vi "GetBarcode 2DResultNames.vi"(7 "ProjectName":string="Prj", 10 "data IN":T1={"ROI"={"Global Rectangle"=[], "Contours"=[]}, "Barcode Type"=enum."PDF417", "Data Matrix Parameter"={"Data Matrix Description Options"={"Aspect Ratio"=0.0, "Rows"=0, "Columns"=0, "Rectangle"=FALSE, "ECC"=-2, "Barcode Polarity"=0, "Cell Fill Percentage"=-2, "Minimum Border Integrity %"=80.0, "Mirror Mode"=-2}, "Data Matrix Search Options"={"Rotation Mode"=enum."Unlimited", "Skip Location?"=FALSE, "Edge Threshold"=30, "Demodulation Mode"=-2, "Cell Sample Size"=-2, "Cell Filter Mode"=-2, "Skew Degrees Allowed"=5, "Maximum Iterations"=500, "Initial Search Vector Width"=5}, "Data Matrix Size Options"={"Data Matrix Size"={"Minimum Size"=0, "Maximum Size"=0}, "Quiet Zone Width"=10}, "Advanced Options"=[]}, "PDF147 Search Mode"=enum."Multiple Barcodes", "QR Code Parameter"={"QR Search Options"={"Rotation Mode"=enum."Unlimited", "Skip Location?"=FALSE, "Edge Threshold"=30, "Demodulation Mode"=-2, "Cell Sample Size"=-2, "Cell Filter Mode"=-2, "Skew Degrees Allowed"=5}, "QR Description Options"={"Matrix Size (cells)"=0, "Barcode Polarity"=-2, "Mirror Mode"=-2, "QR Model"=0}, "QR Code Cell Size (pixels)"={"Minimum Size"=3, "Maximum Size"=7}}} {"QR Code Parameter"."QR Description Options"."Mirror Mode" items=["Auto-detect"=-2, "Normal"=0, "Mirrored"=1]; "QR Code Parameter"."QR Description Options"."Matrix Size (cells)" items=["Auto-detect"=0, "11x11 - Version 1 (Micro QR Only)"=11, "13x13 - Version 2 (Micro QR Only)"=13, "15x15 - Version 3 (Micro QR Only)"=15, "17x17 - Version 4 (Micro QR Only)"=17, "21x21 - Version 1"=21, "25x25 - Version 2"=25, "29x29 - Version 3"=29, "33x33 - Version 4"=33, "37x37 - Version 5"=37, "41x41 - Version 6"=41, "45x45 - Version 7"=45, "49x49 - Version 8"=49, "53x53 - Version 9"=53, "57x57 - Version 10"=57, "61x61 - Version 11"=61, "65x65 - Version 12"=65, "69x69 - Version 13"=69, "73x73 - Version 14"=73, "77x77 - Version 15"=77, "81x81 - Version 16"=81, "85x85 - Version 17"=85, "89x89 - Version 18"=89, "93x93 - Version 19"=93, "97x97 - Version 20"=97, "101x101 - Version 21"=101, "105x105 - Version 22"=105, "109x109 - Version 23"=109, "113x113 - Version 24"=113, "117x117 - Version 25"=117, "121x121 - Version 26"=121, "125x125 - Version 27"=125, "129x129 - Version 28"=129, "133x133 - Version 29"=133, "137x137 - Version 30"=137, "141x141 - Version 31"=141, "145x145 - Version 32"=145, "149x149 - Version 33"=149, "153x153 - Version 34"=153, "157x157 - Version 35"=157, "161x161 - Version 36"=161, "165x165 - Version 37"=165, "169x169 -  Version 38"=169, "173x173 - Version 39"=173, "177x177 - Version 40"=177]; "QR Code Parameter"."QR Description Options"."QR Model" items=["Auto-detect", "Micro", "Model 1", "Model 2"]; "QR Code Parameter"."QR Description Options"."Barcode Polarity" items=["Auto-detect"=-2, "Black on White"=0, "White on Black"=1]; "QR Code Parameter"."QR Search Options"."Cell Filter Mode" items=["Auto-detect"=-2, "Average"=0, "Median"=1, "Central Average"=2, "High Average"=3, "Low Average"=4, "Very High Average"=5, "Very Low Average"=6, "All Filters"=8]; "QR Code Parameter"."QR Search Options"."Cell Sample Size" items=["Auto-detect"=-2, "1x1"=1, "2x2"=2, "3x3"=3, "4x4"=4, "5x5"=5, "6x6"=6, "7x7"=7]; "QR Code Parameter"."QR Search Options"."Demodulation Mode" items=["Auto-detect"=-2, "Histogram"=0, "Local Contrast"=1, "Combination"=2, "All"=3]; "Data Matrix Parameter"."Advanced Options"."Value" format="%.2f"; "Data Matrix Parameter"."Data Matrix Search Options"."Cell Filter Mode" items=["Auto-detect"=-2, "Average"=0, "Median"=1, "Central Average"=2, "High Average"=3, "Low Average"=4, "Very High Average"=5, "Very Low Average"=6, "All Filters"=8]; "Data Matrix Parameter"."Data Matrix Search Options"."Cell Sample Size" items=["Auto-detect"=-2, "1x1"=1, "2x2"=2, "3x3"=3, "4x4"=4, "5x5"=5, "6x6"=6, "7x7"=7]; "Data Matrix Parameter"."Data Matrix Search Options"."Demodulation Mode" items=["Auto-detect"=-2, "Histogram"=0, "Local Contrast"=1, "Combination"=2, "All"=3]; "Data Matrix Parameter"."Data Matrix Description Options"."Mirror Mode" items=["Auto-detect"=-2, "Normal"=0, "Mirrored"=1]; "Data Matrix Parameter"."Data Matrix Description Options"."ECC" items=["Auto-detect"=-2, "ECC 000"=0, "ECC 050"=50, "ECC 080"=80, "ECC 100"=100, "ECC 140"=140, "ECC 000-140"=190, "ECC 200"=200]; "Data Matrix Parameter"."Data Matrix Description Options"."Minimum Border Integrity %" format="%.2f"; "Data Matrix Parameter"."Data Matrix Description Options"."Aspect Ratio" format="%.2f"; "Data Matrix Parameter"."Data Matrix Description Options"."Cell Fill Percentage" items=["Auto-detect"=-2, "< 30%"=0, ">= 30%"=1]; "Data Matrix Parameter"."Data Matrix Description Options"."Barcode Polarity" items=["Auto-detect"=-2, "Black on White"=0, "White on Black"=1]}, 11 "ROI_Name":string="ROI1") -> (3 "ResultNames":string[](array[string]))   [LabVIEW 2019]
uses:
  Controls/Barcode 2D/Analysis_Barcode 2D_Result.ctl
  <vilib>/vision/Instrument.llb/QR Code Report.ctl
  <vilib>/vision/Instrument.llb/QR Code Model Type.ctl
  <vilib>/vision/Instrument.llb/QR Code Stream Mode Type.ctl
  <vilib>/vision/Instrument.llb/Data Matrix Polarity.ctl
  <vilib>/vision/Instrument.llb/Demodulation Mode.ctl
  <vilib>/vision/Instrument.llb/Cell Sample Size.ctl
  <vilib>/vision/Instrument.llb/Cell Filter Mode.ctl
  Controls/Barcode 2D/Analysis_Barcode 2D_Parameter.ctl
  <vilib>/vision/Instrument.llb/Data Matrix Description Options.ctl
  <vilib>/vision/Instrument.llb/ECC Type.ctl
  <vilib>/vision/Instrument.llb/Cell Fill Percentage.ctl
  <vilib>/vision/Instrument.llb/Data Matrix Mirror.ctl
  <vilib>/vision/Instrument.llb/Data Matrix Search Options.ctl
  <vilib>/vision/Instrument.llb/Data Matrix Size Options.ctl
  <vilib>/vision/Instrument.llb/Data Matrix Advanced Options.ctl
  <vilib>/vision/Instrument.llb/QR Code Search Options.ctl
  <vilib>/vision/Instrument.llb/QR Code Description Options.ctl
panel:
  out "Analysis_Barcode 2D_Result":T17={"QR Code Report"={"Found?"=FALSE, "Data"="", "Bounding Box"=[], "Errors Corrected"=0, "Dimensions (Rows/Cols)"=0, "Version"=0, "QR Model"=0, "Stream Mode"=0, "Barcode Polarity"=-2, "Mirrored?"=FALSE, "Append Stream Position"=0, "Size of Append Stream"=0, "First EAN-128 ID"=0, "First Alternate Language ID"=0, "Append Stream ID"=0, "Minimum Edge Strength"=30, "Demodulation Mode"=-2, "Cell Sample Size"=-2, "Cell Filter Mode"=-2}} {"QR Code Report"."Append Stream ID" format="%x"; "QR Code Report"."Cell Filter Mode" items=["Auto-detect"=-2, "Average"=0, "Median"=1, "Central Average"=2, "High Average"=3, "Low Average"=4, "Very High Average"=5, "Very Low Average"=6, "All Filters"=8]; "QR Code Report"."Cell Sample Size" items=["Auto-detect"=-2, "1x1"=1, "2x2"=2, "3x3"=3, "4x4"=4, "5x5"=5, "6x6"=6, "7x7"=7]; "QR Code Report"."Demodulation Mode" items=["Auto-detect"=-2, "Histogram"=0, "Local Contrast"=1, "Combination"=2, "All"=3]; "QR Code Report"."Barcode Polarity" items=["Auto-detect"=-2, "Black on White"=0, "White on Black"=1]; "QR Code Report"."Stream Mode" items=["Numeric", "AlphaNumeric", "Raw Bytes", "UCC/EAN-128 - In Tokens", "UCC/EAN-128 - In Data", "Extended Character Interpretation", "Kanji"]; "QR Code Report"."QR Model" items=["Auto-detect", "Micro", "Model 1", "Model 2"]; "QR Code Report"."Version" max=40 step=1}
  out "error out":errorcluster
  in  "error in (no error)":errorcluster
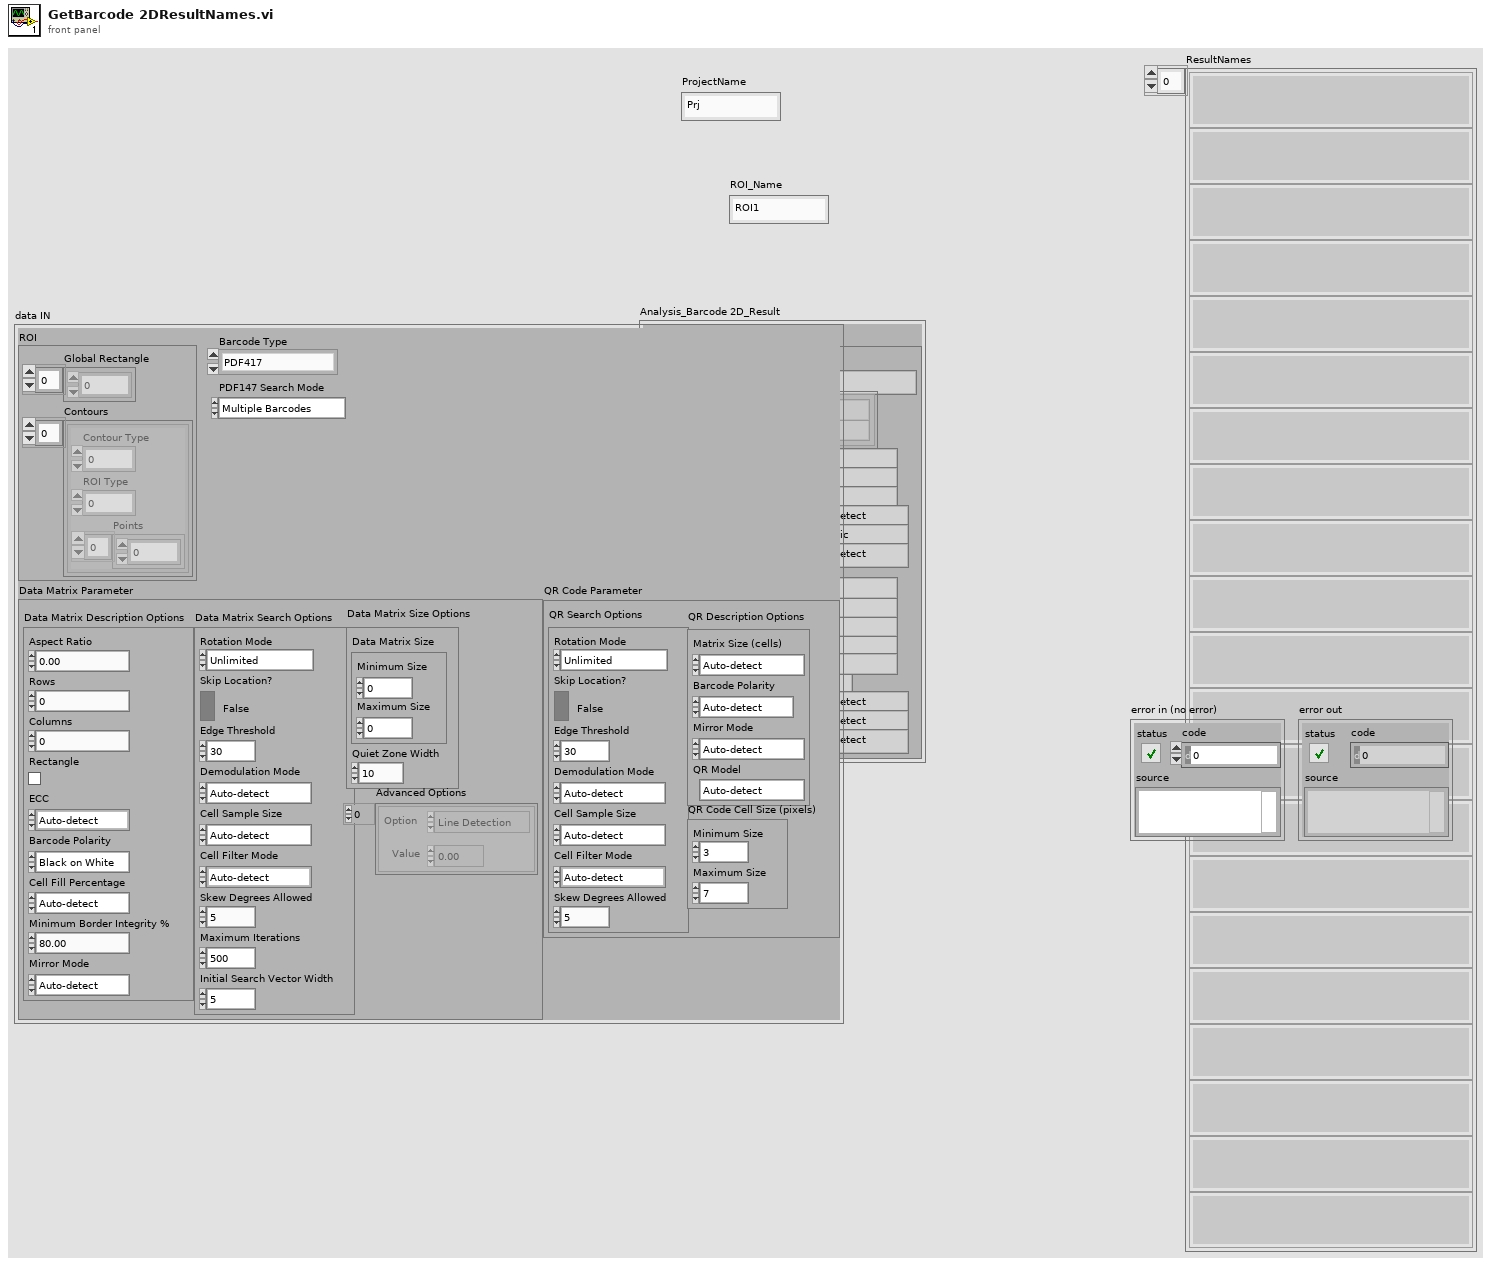
[diagram p1: front panel]
types:
  T1 = typedef "Analysis_Barcode 2D_Parameter.ctl" = cluster{"ROI":cluster{"Global Rectangle":i32[], "Contours":cluster{"Contour Type":u32, "ROI Type":u32, "Points":i32[]}[]}, "Barcode Type":enum16{"Data Matrix", "PDF417", "QR Code"}, "Data Matrix Parameter":cluster{"Data Matrix Description Options":T2, "Data Matrix Search Options":T7, "Data Matrix Size Options":T11, "Advanced Options":T12[]}, "PDF147 Search Mode":T13, "QR Code Parameter":cluster{"QR Search Options":T14, "QR Description Options":T15, "QR Code Cell Size (pixels)":cluster{"Minimum Size":u32, "Maximum Size":u32}}}
  T2 = typedef "Data Matrix Description Options.ctl" = cluster{"Aspect Ratio":sgl, "Rows":u32, "Columns":u32, "Rectangle":bool, "ECC":T3, "Barcode Polarity":T4, "Cell Fill Percentage":T5, "Minimum Border Integrity %":sgl, "Mirror Mode":T6}
  T3 = typedef "ECC Type.ctl" = i32
  T4 = typedef "Data Matrix Polarity.ctl" = i32
  T5 = typedef "Cell Fill Percentage.ctl" = i32
  T6 = typedef "Data Matrix Mirror.ctl" = i32
  T7 = typedef "Data Matrix Search Options.ctl" = cluster{"Rotation Mode":enum32{"Unlimited", "0 Degrees", "90 Degrees", "180 Degrees", "270 Degrees"}, "Skip Location?":bool, "Edge Threshold":u32, "Demodulation Mode":T8, "Cell Sample Size":T9, "Cell Filter Mode":T10, "Skew Degrees Allowed":u32, "Maximum Iterations":u32, "Initial Search Vector Width":u32}
  T8 = typedef "Demodulation Mode.ctl" = i32
  T9 = typedef "Cell Sample Size.ctl" = i32
  T10 = typedef "Cell Filter Mode.ctl" = i32
  T11 = typedef "Data Matrix Size Options.ctl" = cluster{"Data Matrix Size":cluster{"Minimum Size":u32, "Maximum Size":u32}, "Quiet Zone Width":u32}
  T12 = typedef "Data Matrix Advanced Options.ctl" = cluster{"Option":enum32{"Line Detection", "HighLight Filter", "Aggressive", "FNC1", "Refine Bounding Box"}, " Value":dbl}
  T13 = typedef "PDF417 Search Mode" = enum32{"Multiple Barcodes", "Single Barcode, Conservative"}
  T14 = typedef "QR Code Search Options.ctl" = cluster{"Rotation Mode":enum32{"Unlimited", "0 Degrees", "90 Degrees", "180 Degrees", "270 Degrees"}, "Skip Location?":bool, "Edge Threshold":u32, "Demodulation Mode":T8, "Cell Sample Size":T9, "Cell Filter Mode":T10, "Skew Degrees Allowed":u32}
  T15 = typedef "QR Code Description Options.ctl" = cluster{"Matrix Size (cells)":i32, "Barcode Polarity":T4, "Mirror Mode":i32, "QR Model":T16}
  T16 = typedef "QR Code Model Type.ctl" = i32
  T17 = typedef "Analysis_Barcode 2D_Result.ctl" = cluster{"QR Code Report":T18}
  T18 = typedef "QR Code Report.ctl" = cluster{"Found?":bool, "Data":string, "Bounding Box":cluster{"x":sgl, "y":sgl}[], "Errors Corrected":u32, "Dimensions (Rows/Cols)":u32, "Version":u32, "QR Model":T16, "Stream Mode":T19, "Barcode Polarity":T4, "Mirrored?":bool, "Append Stream Position":u32, "Size of Append Stream":u32, "First EAN-128 ID":i32, "First Alternate Language ID":i32, "Append Stream ID":u32, "Minimum Edge Strength":u32, "Demodulation Mode":T8, "Cell Sample Size":T9, "Cell Filter Mode":T10}
  T19 = typedef "QR Code Stream Mode Type.ctl" = i32
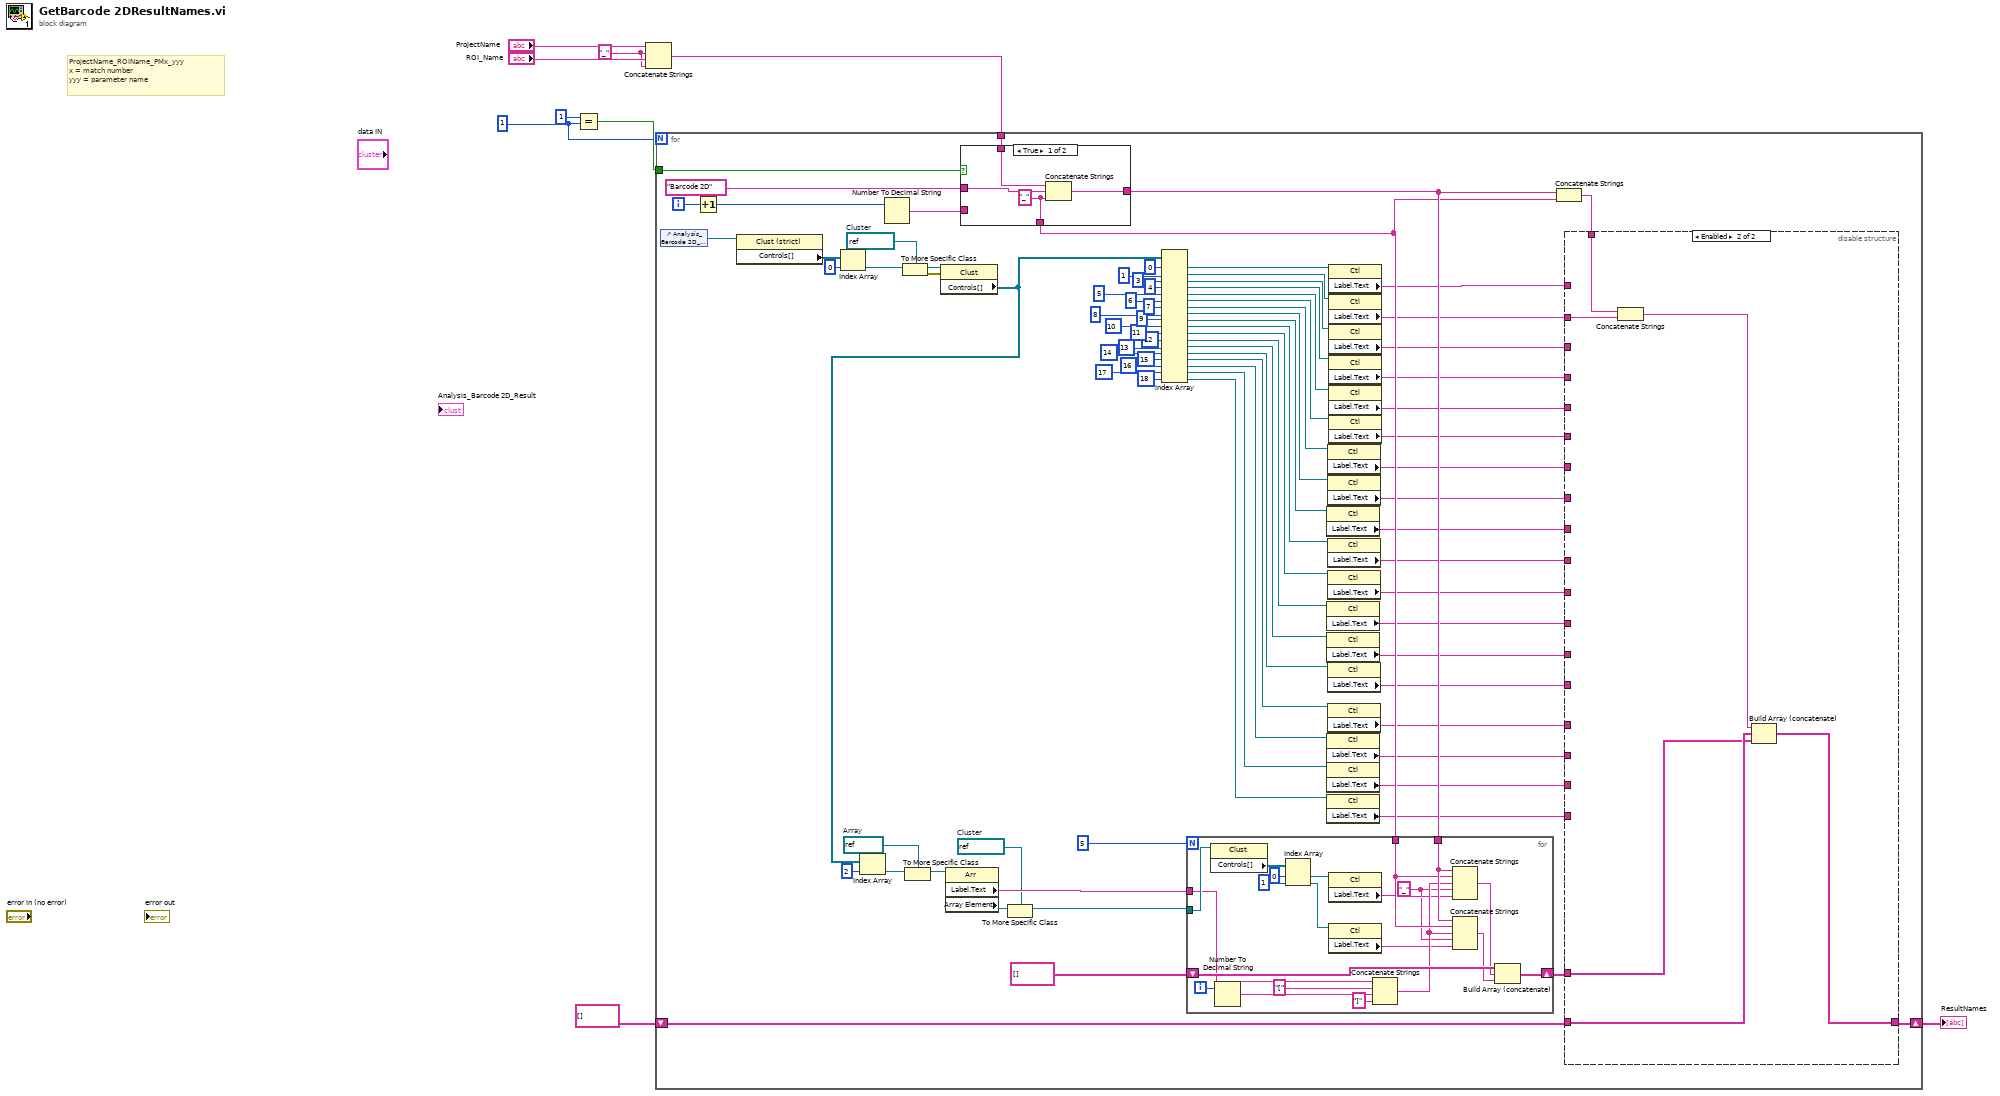
[diagram p0: block diagram]
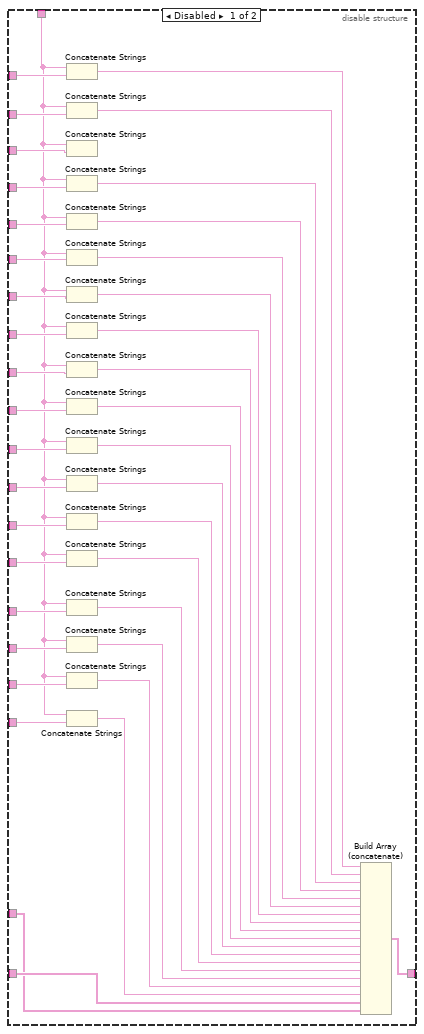
[diagram p2: hidden frame]
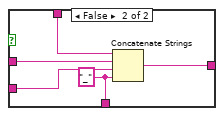
[diagram p3: hidden frame]
diagram:
  w1 = 1
  w6 = "_" ("string")
  # "ProjectName_ROIName_PMx_yyy\nx = match number\nyyy = parameter name"
  n1 = Equal?(x=1, y=w1) -> (x = y?=w2:bool)
  n2 = Concatenate Strings("ProjectName", w6, "ROI_Name", w6) -> (w5:string)
  n3 = for {
    N: w1 -> [_]
    tunnel: w5 -> [w91]
    shift-right: [w64] -> w3
    shift-left: string[] [] -> [w87]
    tunnel: w2 -> [w92]
    i -> [w88]
    w52 = refnum<vi> refnum  # Cluster
    w54 = refnum<vi> refnum  # Array
    w57 = refnum<vi> refnum  # Cluster
    n4 = control-ref of="Analysis_Barcode 2D_Result"() -> (w61:refnum<vi>)
    n5 = Increment(x=w88) -> (x+1=w93:i32)
    n6 = property class="Clust (strict)"(reference=w61) -> ("Controls[]"=w60:refnum<vi>[])  [unwired: 1 in, 2 out]
    n7 = Index Array(array=w60, index=0) -> (element=w58:refnum<vi>)
    n8 = Number To Decimal String(number=w93) -> (decimal integer string=w90:string)  [unwired: 1 in]
    n9 = To More Specific Class(target class=w57, reference=w58) -> (specific class reference=w56:refnum<vi>, error out=w55:errorcluster)  [unwired: 1 in]
    n10 = property class="Clust"(reference=w56, error in=w55) -> ("Controls[]"=w48:refnum<vi>[])  [unwired: 2 out]
    n11 = Index Array(array=w48, index=2) -> (element=w50:refnum<vi>)
    n12 = To More Specific Class(target class=w54, reference=w50) -> (specific class reference=w53:refnum<vi>)  [unwired: 1 in, 1 out]
    n13 = property class="Arr"(reference=w53) -> ("Label.Text"=w86:string, "Array Element"=w51:refnum<vi>)  [unwired: 1 in, 2 out]
    n14 = case shown="True" w92 {
      tunnel: w91 -> [w163 w168]
      tunnel: w90 -> [_ w166]
      tunnel: [w162 w167] -> w71
      tunnel: "Barcode 2D" ("string") -> [w161 w165]
      tunnel: [w160 w164] -> w70
      frame True {
        w160 = "_" ("string")
        n15 = Concatenate Strings(w163, w161, w160) -> (w162:string)
      }
      frame False {
        w164 = "_" ("string")
        n16 = Concatenate Strings(w168, w165, w166, w164) -> (w167:string)
      }
    }
    n17 = To More Specific Class(target class=w52, reference=w51) -> (specific class reference=w82:refnum<vi>)  [unwired: 1 in, 1 out]
    n18 = Index Array(array=w48, index #1=0 ("index"), index #2=1 ("index"), index #3=3 ("index"), index #4=4 ("index"), index #5=5 ("index"), index #6=6, index #7=7 ("index"), index #8=8 ("index"), index #9=9, index #10=10 ("index"), index #11=11 ("index"), index #12=12 ("index"), index #13=13 ("index"), index #14=14 ("index"), index #15=15 ("index"), index #16=16 ("index"), index #17=17 ("index"), index #18=18 ("index")) -> (element #1=w77:refnum<vi>, element #2=w76:refnum<vi>, element #3=w75:refnum<vi>, element #4=w74:refnum<vi>, element #5=w72:refnum<vi>, element #6=w63:refnum<vi>, element #7=w43:refnum<vi>, element #8=w42:refnum<vi>, element #9=w38:refnum<vi>, element #10=w36:refnum<vi>, element #11=w35:refnum<vi>, element #12=w34:refnum<vi>, element #13=w33:refnum<vi>, element #14=w32:refnum<vi>, element #15=w31:refnum<vi>, element #16=w30:refnum<vi>, element #17=w20:refnum<vi>, element #18=w19:refnum<vi>)
    n19 = for {
      N: 5 -> [_]
      tunnel: w86 -> [w151]
      tunnel: w82 -> [w159]
      tunnel: w71 -> [w158]
      tunnel: w70 -> [w157]
      shift-right: [w153] -> w83
      shift-left: string[] [] -> [w156]
      i -> [w152]
      w145 = "_" ("string")
      n20 = property class="Clust"(reference=w159) -> ("Controls[]"=w144:refnum<vi>[])  [unwired: 1 in, 2 out]
      n21 = Number To Decimal String(number=w152) -> (decimal integer string=w149:string)  [unwired: 1 in]
      n22 = Index Array(array=w144, index #1=0 ("index"), index #2=1 ("index")) -> (element #1=w142:refnum<vi>, element #2=w139:refnum<vi>)
      n23 = property class="Ctl"(reference=w142) -> ("Label.Text"=w146:string)  [unwired: 1 in, 2 out]
      n24 = property class="Ctl"(reference=w139) -> ("Label.Text"=w140:string)  [unwired: 1 in, 2 out]
      n25 = Concatenate Strings(w151, "[" ("string"), w149, "]" ("string")) -> (w147:string)
      n26 = Concatenate Strings(w158, w157, w147, w145, w146) -> (w155:string)
      n27 = Concatenate Strings(w158, w157, w147, w145, w140) -> (w154:string)
      n28 = Build Array (concatenate)(w156, w155, w154) -> (w153:string[])
    }
    n29 = property class="Ctl"(reference=w38) -> ("Label.Text"=w37:string)  [unwired: 1 in, 2 out]
    n30 = property class="Ctl"(reference=w34) -> ("Label.Text"=w16:string)  [unwired: 1 in, 2 out]
    n31 = property class="Ctl"(reference=w33) -> ("Label.Text"=w15:string)  [unwired: 1 in, 2 out]
    n32 = property class="Ctl"(reference=w30) -> ("Label.Text"=w12:string)  [unwired: 1 in, 2 out]
    n33 = property class="Ctl"(reference=w20) -> ("Label.Text"=w11:string)  [unwired: 1 in, 2 out]
    n34 = property class="Ctl"(reference=w19) -> ("Label.Text"=w10:string)  [unwired: 1 in, 2 out]
    n35 = property class="Ctl"(reference=w43) -> ("Label.Text"=w41:string)  [unwired: 1 in, 2 out]
    n36 = property class="Ctl"(reference=w42) -> ("Label.Text"=w40:string)  [unwired: 1 in, 2 out]
    n37 = property class="Ctl"(reference=w36) -> ("Label.Text"=w18:string)  [unwired: 1 in, 2 out]
    n38 = property class="Ctl"(reference=w35) -> ("Label.Text"=w17:string)  [unwired: 1 in, 2 out]
    n39 = property class="Ctl"(reference=w32) -> ("Label.Text"=w14:string)  [unwired: 1 in, 2 out]
    n40 = property class="Ctl"(reference=w31) -> ("Label.Text"=w13:string)  [unwired: 1 in, 2 out]
    n41 = property class="Ctl"(reference=w77) -> ("Label.Text"=w69:string)  [unwired: 1 in, 2 out]
    n42 = property class="Ctl"(reference=w76) -> ("Label.Text"=w68:string)  [unwired: 1 in, 2 out]
    n43 = property class="Ctl"(reference=w75) -> ("Label.Text"=w46:string)  [unwired: 1 in, 2 out]
    n44 = property class="Ctl"(reference=w74) -> ("Label.Text"=w67:string)  [unwired: 1 in, 2 out]
    n45 = property class="Ctl"(reference=w72) -> ("Label.Text"=w66:string)  [unwired: 1 in, 2 out]
    n46 = property class="Ctl"(reference=w63) -> ("Label.Text"=w62:string)  [unwired: 1 in, 2 out]
    n47 = Concatenate Strings(w71, w70) -> (w65:string)
    n48 = disable-structure shown="Enabled" {
      disable-tunnel: w87 -> [w132 w138]
      disable-tunnel: w83 -> [w131 w137]
      disable-tunnel: w69 -> [w130 _]
      disable-tunnel: w68 -> [w129 w135]
      disable-tunnel: w67 -> [w128 _]
      disable-tunnel: w66 -> [w127 _]
      disable-tunnel: w65 -> [w106 w134]
      disable-tunnel: [w123 w136] -> w64
      disable-tunnel: w62 -> [w121 _]
      disable-tunnel: w46 -> [w119 _]
      disable-tunnel: w41 -> [w118 _]
      disable-tunnel: w40 -> [w117 _]
      disable-tunnel: w37 -> [w116 _]
      disable-tunnel: w18 -> [w115 _]
      disable-tunnel: w17 -> [w114 _]
      disable-tunnel: w16 -> [w113 _]
      disable-tunnel: w15 -> [w112 _]
      disable-tunnel: w14 -> [w111 _]
      disable-tunnel: w13 -> [w110 _]
      disable-tunnel: w12 -> [w109 _]
      disable-tunnel: w11 -> [w108 _]
      disable-tunnel: w10 -> [w107 _]
      frame Disabled {
        n49 = Concatenate Strings(w106, w130) -> (w126:string)
        n50 = Concatenate Strings(w106, w129) -> (w125:string)
        n51 = Concatenate Strings(w106, w119) -> ()  [unwired: 1 out]
        n52 = Concatenate Strings(w106, w128) -> (w124:string)
        n53 = Concatenate Strings(w106, w127) -> (w122:string)
        n54 = Concatenate Strings(w106, w121) -> (w120:string)
        n55 = Concatenate Strings(w106, w118) -> (w105:string)
        n56 = Concatenate Strings(w106, w117) -> (w104:string)
        n57 = Concatenate Strings(w106, w116) -> (w103:string)
        n58 = Concatenate Strings(w106, w115) -> (w102:string)
        n59 = Concatenate Strings(w106, w114) -> (w101:string)
        n60 = Concatenate Strings(w106, w113) -> (w100:string)
        n61 = Concatenate Strings(w106, w112) -> (w99:string)
        n62 = Concatenate Strings(w106, w111) -> (w98:string)
        n63 = Concatenate Strings(w106, w110) -> (w97:string)
        n64 = Concatenate Strings(w106, w109) -> (w96:string)
        n65 = Concatenate Strings(w106, w108) -> (w95:string)
        n66 = Concatenate Strings(w106, w107) -> (w94:string)
        n67 = Build Array (concatenate)(w126, w125, w124, w122, w120, w105, w104, w103, w102, w101, w100, w99, w98, w97, w96, w95, w94, w132, w131) -> (w123:string[])
      }
      frame Enabled {
        n68 = Concatenate Strings(w134, w135) -> (w133:string)
        n69 = Build Array (concatenate)(w133, w138, w137) -> (w136:string[])
      }
    }
  }
  "ResultNames" <- w3
